vi "CSClassUtilities.InheritClass.vi"() -> ()   [LabVIEW 2014]
doc: "This tool allows one to inherit a class from a parent class.\n\nLicense Agreement for this software:\n\nCopyright (C) 2001 Dietrich Beck, Holger Brand, Mathias Richter\nGSI Helmholtzzentrum für Schwerionenforschung GmbH\nPlanckstraße 1\nD-64291 Darmstadt\nGermany\n\nContact: d.beck@gsi.de \n\nThis program is free software: you can redistribute it and/or modify it under the terms\nof the GNU General Public License as published by the Free Software Foundation, either\nversion 3 of the License, or (at your option) any later version.\n\nThis program is distributed in the hope that it will be useful, but WITHOUT ANY WARRANTY;\nwithout even the implied warranty of MERCHANTABILITY or FITNESS FOR A PARTICULAR PURPOSE. See the GNU General Public License for more details.\n\nYou should have received a copy of the GNU General Public License along with this program.\nIf not, see <http://www.gnu.org/licenses/>.\n\nFor all questions and ideas contact: d.beck@gsi.de\nLast update: 19-Nov-2010"
uses:
  CSClass/CSCore/CSSystem/CoreLib/CoreLib.lvlib
  CSClass/CSCore/CSSystem/CSSystemLib/CSSystemLib.lvlib
panel:
  in  "GUI":T1(tab)=enum."NewClass"
  in  "Continue1":bool
  in  "Continue2":bool
  in  "Select parent class":i32(listbox)
  in  "Continue3":bool
  in  "New class name":string
  in  "Select Class Group":i32(listbox)
  out "Done?":bool
  out "Parent Class":string
  out "New Class":string
  # "1) This tool  will open and rename a couple of VIs. It is strongly recommended to use this tool not from a project but directly after launching LabVIEW!\n\n2) This tool may overwrite existing VIs. It is recommended to back up the class directory structure.\n\n3) This tool will only work on classes that are below the \".../CSClass\" folder.\n\n4) Public and protected class methods of a class will not be re-created in the child class. If you would like to use such methods of a (grand-) parent class, use direct method calls. No copy and paste! As a consequence, this tool is not required for inheritance. The parent class of a child class is defined by calling the constructor of the parent class within the constructor of the child class (Of course, one should call the deconstructor of the parent class within the deconstructor of the child class).\n\n5) Only in exceptional cases, copies of methods must be created in a child class.  Examples are the constructor/destructor methods.. \n\nPLEASE CONTINUE ONLY, IF THIS VI HAS BEEN LOADED DIRECTLY AFTER LAUNCHING LabVIEW!"
  # "1) When done, it is recommended to exit and restart LabVIEW.\n\n2) It is good idea to refine the methods of the class created by \n     a) modifying the icons of the methods.\n     b) editing the attribute data (.../CLASSNAME/private/i attribute.ctl).\n     c) adding new functionality to the class."
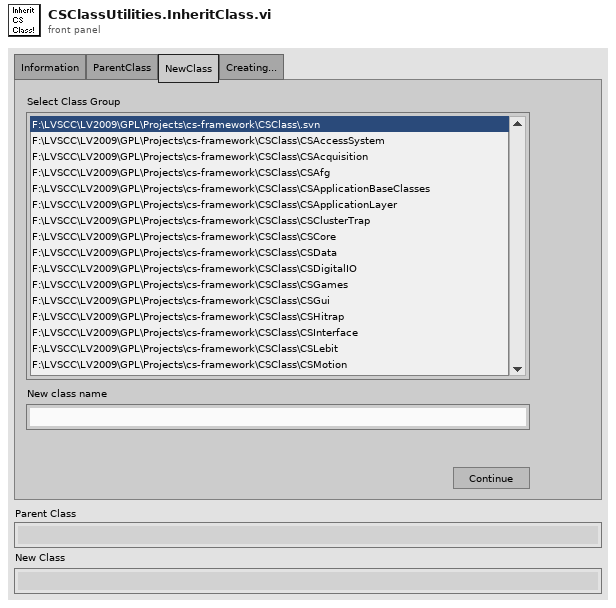
[diagram p1: front panel]
types:
  T1 = enum32{"Information", "ParentClass", "NewClass", "Creating..."}
  T2 = enum32{"invalid scope", "public", "private", "protected"}
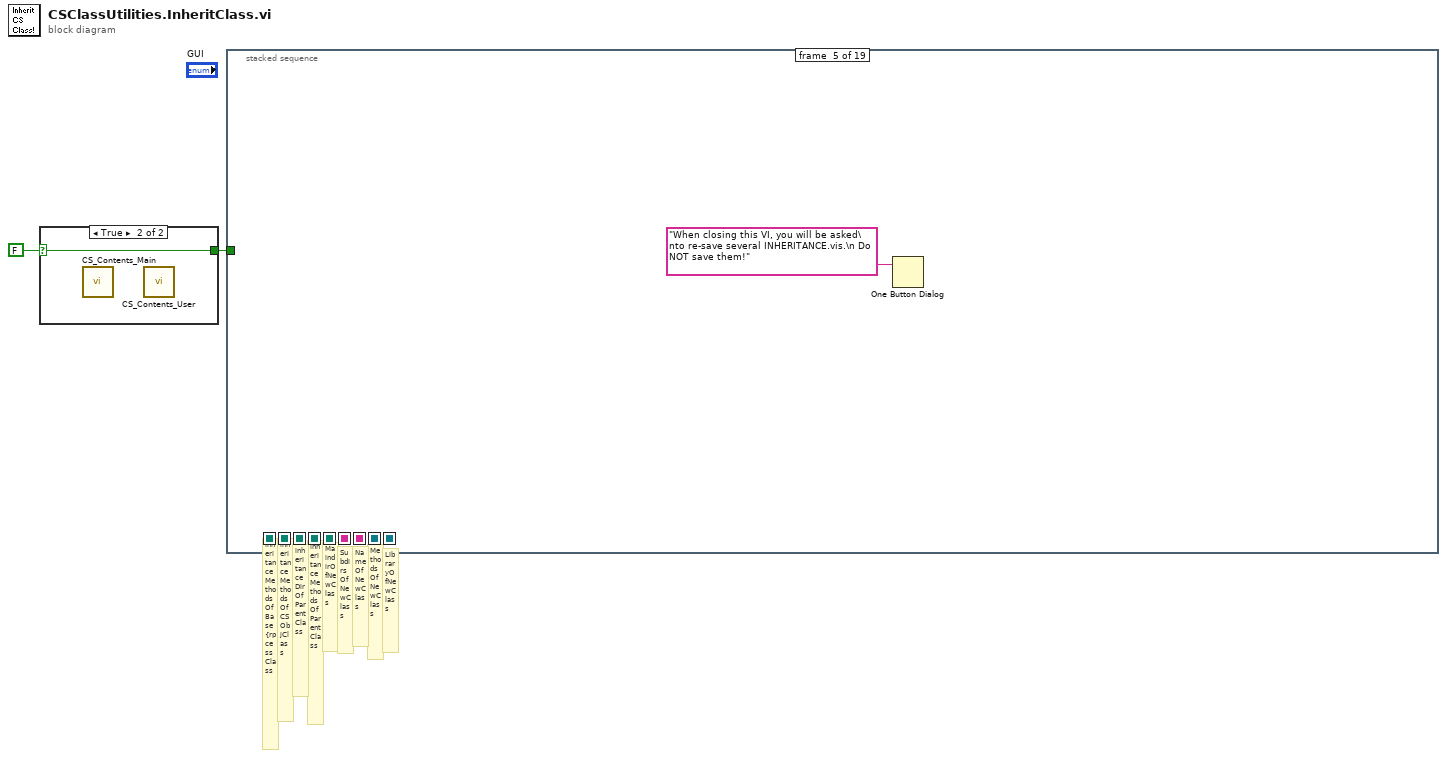
[diagram p0: block diagram]
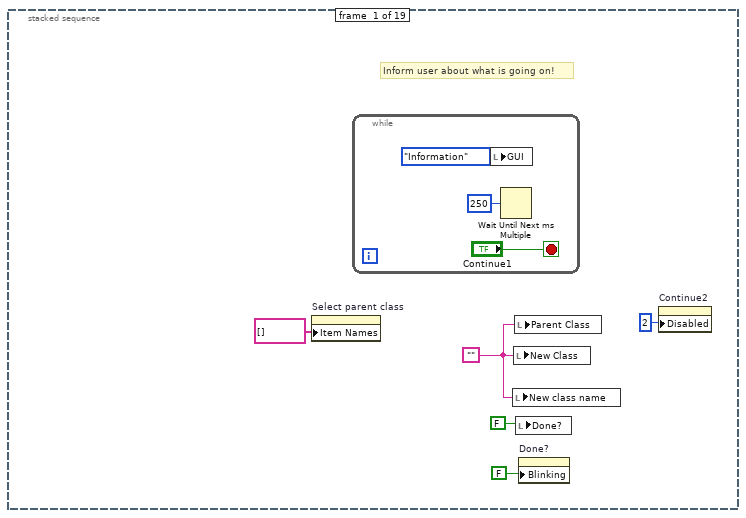
[diagram p3: hidden frame]
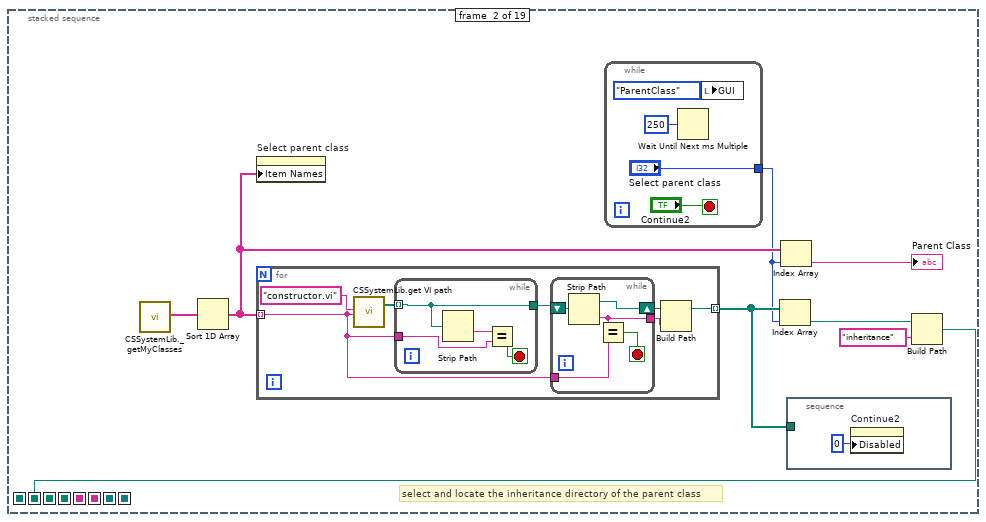
[diagram p4: hidden frame]
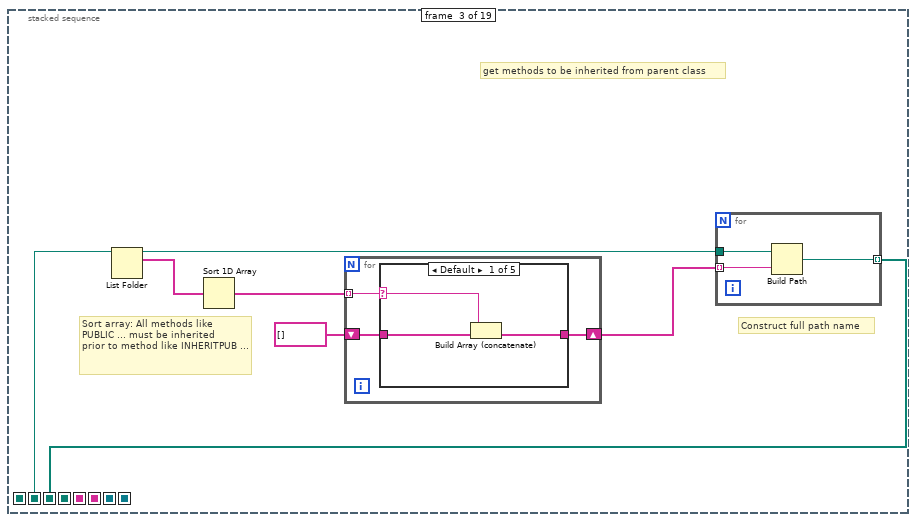
[diagram p5: hidden frame]
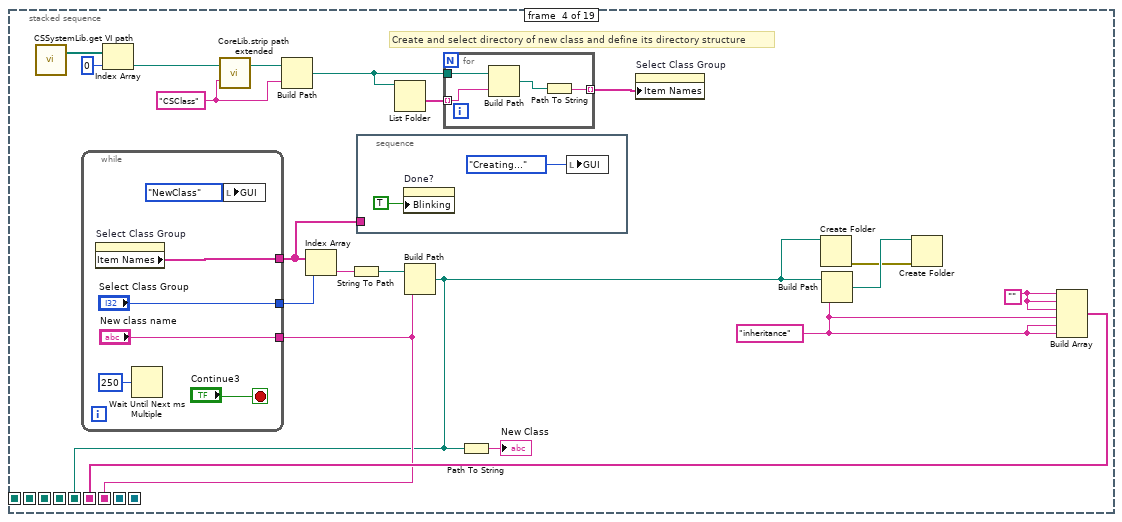
[diagram p10: hidden frame]
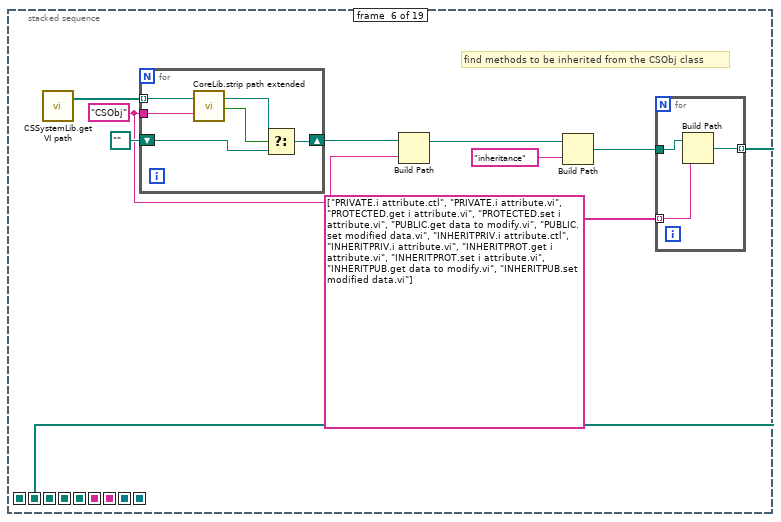
[diagram p11: hidden frame]
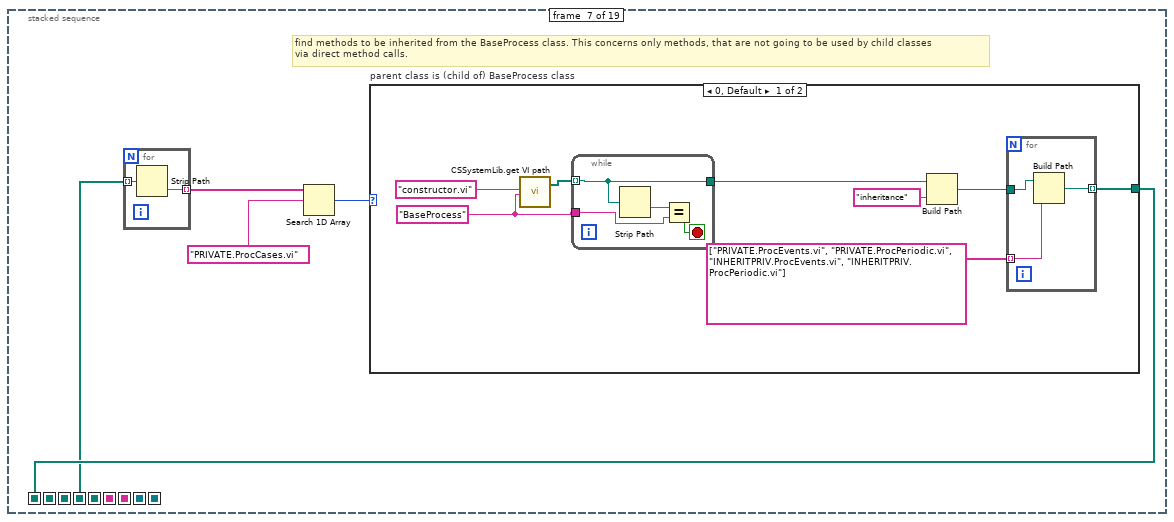
[diagram p12: hidden frame]
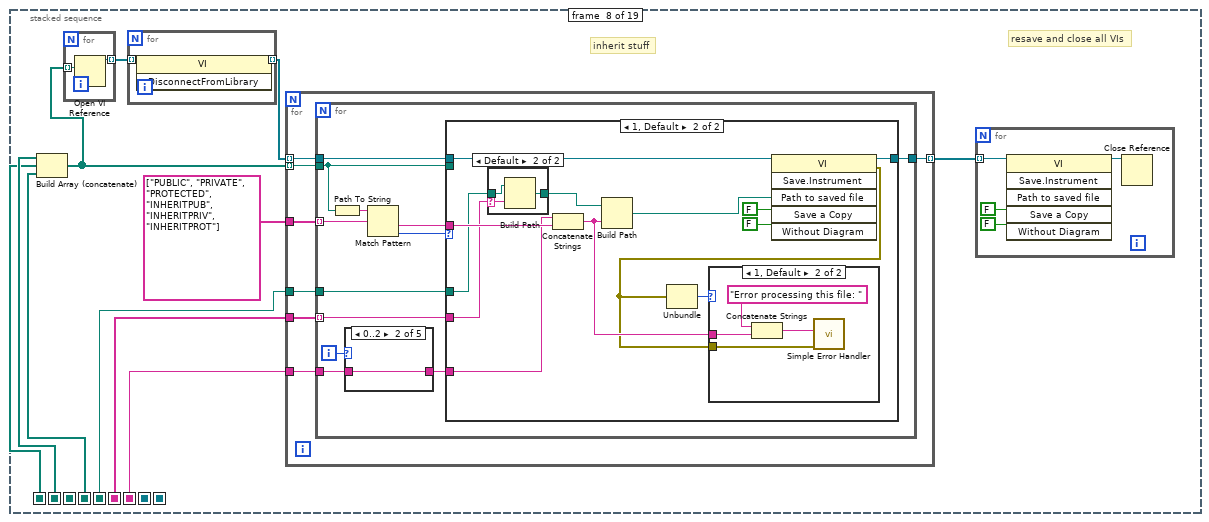
[diagram p14: hidden frame]
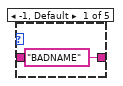
[diagram p15: hidden frame]
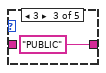
[diagram p16: hidden frame]
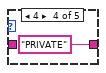
[diagram p17: hidden frame]
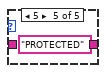
[diagram p18: hidden frame]
diagram:
  # "LibraryOfNewClass"
  # "MethodsOfNewClass"
  # "inheritanceMethodsOfBase{rpcessClass"
  # "inheritanceMethodsOfCSObjClass"
  # "NameOfNewClass"
  # "MaindirOfNewClass"
  # "SubdirsOfNewClass"
  # "inheritanceMethodsOfParentClass"
  # "inheritanceDirOfParentClass"
  n1 = case shown="True" FALSE {
    selector: FALSE -> [_ w3]
    tunnel: [_ w3] -> w1
    frame False {
    }
    frame True {
      n2 = call "CS_Contents_Main.vi"() -> ()  [unwired: 1 in]
      n3 = call "CS_Contents_User.vi"() -> ()  [unwired: 1 in]
    }
  }
  n4 = stacked-sequence {
    seq-local: [_ _ _ w67 _ _ _ _ _ _ _ _ _ _ _ _ _ _ _] -> [_ _ _ _ _ _ _ w144 _ _ _ _ w274 w305 w334 w362 w400 _ _]
    seq-local: [_ _ _ w77 _ _ _ _ _ _ _ _ _ _ _ _ _ _ _] -> [_ _ _ _ _ _ _ w143 _ _ _ _ _ _ _ _ _ _ _]
    seq-local: [_ w19 _ _ _ _ _ _ _ _ _ _ _ _ _ _ _ _ _] -> [_ _ w47 _ _ _ _ _ _ _ _ _ _ _ _ _ _ _ _]
    seq-local: [_ _ w44 _ _ _ _ _ _ _ _ _ _ _ _ _ _ _ _] -> [_ _ _ _ _ _ w114 w139 w200 w222 _ _ _ _ _ _ _ _ _]
    seq-local: [_ _ _ w66 _ _ _ _ _ _ _ _ _ _ _ _ _ _ _] -> [_ _ _ _ _ _ _ w134 w199 w221 w243 w260 w273 w304 w333 w361 w401 _ _]
    seq-local: [_ _ _ _ _ w97 _ _ _ _ _ _ _ _ _ _ _ _ _] -> [_ _ _ _ _ _ _ w140 _ _ _ _ _ _ _ _ _ _ _]
    seq-local: [_ _ _ _ _ _ w116 _ _ _ _ _ _ _ _ _ _ _ _] -> [_ _ _ _ _ _ _ w138 _ _ _ _ _ _ _ _ _ _ _]
    seq-local: [_ _ _ _ _ _ _ _ _ _ _ w250 _ _ _ _ _ _ _] -> [_ _ _ _ _ _ _ _ _ _ _ _ _ _ _ _ _ w403 _]
    seq-local: [_ _ _ _ _ _ _ _ _ _ _ _ w269 _ _ _ _ _ _] -> [_ _ _ _ _ _ _ _ _ _ _ _ _ w301 w330 w358 w394 _ _]
    tunnel: w1 -> [_ _ _ _ _ _ _ _ _ _ _ _ _ _ _ _ _ _ _]
    frame #0 {
      w6 = "" ("New class name")
      # "Inform user about what is going on!"
      n5 = property on="Select parent class" class="LstBox (strict)"("Item Names"=string[] []) -> ()  [unwired: 2 in, 2 out]
      n6 = while {
        stop <- "Continue1" stop-if-true
        n7 = local write "GUI"(T1."Information" ("GUI")) -> ()
        n8 = Wait Until Next ms Multiple(millisecond multiple=u32 250) -> ()  [unwired: 1 out]
      }
      n9 = local write "New class name"(w6) -> ()
      n10 = local write "New Class"(w6) -> ()
      n11 = local write "Parent Class"(w6) -> ()
      n12 = local write "Done?"(FALSE ("Done?")) -> ()
      n13 = property on="Done?" class="Bool (strict)"("Blinking"=FALSE) -> ()  [unwired: 2 in, 2 out]
      n14 = property on="Continue2" class="Bool"("Disabled"=u8 2) -> ()  [unwired: 2 in, 2 out]
    }
    frame #1 {
      # "select and locate the inheritance directory of the parent class"
      n15 = call "CSSystemLib._getMyClasses.vi"() -> ("myClasses"=w16:string[])  [unwired: 18 in, 1 out]
      n16 = Sort 1D Array(array=w16) -> (sorted array=w14:string[])
      n17 = property on="Select parent class" class="LstBox (strict)"("Item Names"=w14) -> ()  [unwired: 2 in, 2 out]
      n18 = for {
        tunnel: w14 -> [w20] mode=indexing
        tunnel: [w23] -> w15 mode=indexing
        n19 = call "CSSystemLib.get VI path.vi"("method"="constructor.vi" ("Method"), "class"=w20) -> ("Directories"=w22:path[])  [unwired: 15 in, 2 out]
        n20 = while {
          tunnel: w22 -> [w29] mode=indexing
          tunnel: [w29] -> w21
          tunnel: w20 -> [w28]
          stop <- w27 stop-if-true
          n21 = Strip Path(path=w29) -> (name=w30:string)  [unwired: 1 out]
          n22 = Equal?(x=w30, y=w28) -> (x = y?=w27:bool)
        }
        n23 = while {
          shift-right: [w34] -> w25
          shift-left: w21 -> [w35]
          tunnel: w20 -> [w33]
          tunnel: [w31] -> w24
          stop <- w32 stop-if-true
          n24 = Strip Path(path=w35) -> (stripped path=w34:path, name=w31:string)
          n25 = Equal?(x=w31, y=w33) -> (x = y?=w32:bool)
        }
        n26 = Build Path(base path=w25, name or relative path=w24) -> (appended path=w23:path)
      }
      n27 = while {
        tunnel: ["Select parent class"] -> w13
        stop <- "Continue2" stop-if-true
        n28 = Wait Until Next ms Multiple(millisecond multiple=u32 250) -> ()  [unwired: 1 out]
        n29 = local write "GUI"(T1."ParentClass" ("GUI")) -> ()
      }
      n30 = Index Array(array=w15, index=w13) -> (element=w17:path)
      n31 = Index Array(array=w14, index=w13) -> (element=→"Parent Class":string)
      n32 = stacked-sequence {
        tunnel: w15 -> [_]
        frame #0 {
          n33 = property on="Continue2" class="Bool"("Disabled"=u8 0) -> ()  [unwired: 2 in, 2 out]
        }
      }
      n34 = Build Path(base path=w17, name or relative path="inheritance") -> (appended path=w19:path)
    }
    frame #2 {
      # "get methods to be inherited from parent class"
      # "Construct full path name"
      # "Sort array: All methods like\nPUBLIC ... must be inherited\nprior to method like INHERITPUB ..."
      n35 = List Folder(path=w47) -> (path out=w45:path, filenames=w46:string[])  [unwired: 3 in, 2 out]
      n36 = Sort 1D Array(array=w46) -> (sorted array=w42:string[])
      n37 = for {
        tunnel: w42 -> [w50] mode=indexing
        shift-right: [w48] -> w41
        shift-left: string[] [] -> [w49]
        n38 = case shown="Default" w50 {
          selector: w50 -> [w51 _ _ _ _]
          tunnel: w49 -> [w53 w54 w55 w56 w57]
          tunnel: [w52 w54 w55 w56 w57] -> w48
          frame Default {
            n39 = Build Array (concatenate)(w51, w53) -> (w52:string[])
          }
          frame "PRIVATE.ProcEvents.vi" {
          }
          frame "PRIVATE.ProcPeriodic.vi" {
          }
          frame "INHERITPRIV.ProcEvents.vi" {
          }
          frame "INHERITPRIV.ProcPeriodic.vi" {
          }
        }
      }
      n40 = for {
        tunnel: w41 -> [w59] mode=indexing
        tunnel: w45 -> [w60]
        tunnel: [w58] -> w44 mode=indexing
        n41 = Build Path(base path=w60, name or relative path=w59) -> (appended path=w58:path)
      }
    }
    frame #3 {
      w62 = "" ("Empty String Constant")
      w63 = "inheritance"
      w71 = "CSClass" ("search string")
      # "Create and select directory of new class and define its directory structure"
      n42 = call "CSSystemLib.get VI path.vi"() -> ("Directories"=w79:path[])  [unwired: 17 in, 2 out]
      n43 = while {
        tunnel: [w90] -> w76
        tunnel: ["Select Class Group"] -> w78
        tunnel: ["New class name"] -> w67
        stop <- "Continue3" stop-if-true
        n44 = property on="Select Class Group" class="LstBox (strict)"() -> ("Item Names"=w90:string[])  [unwired: 2 in, 2 out]
        n45 = Wait Until Next ms Multiple(millisecond multiple=u32 250) -> ()  [unwired: 1 out]
        n46 = local write "GUI"(T1."NewClass" ("GUI")) -> ()
      }
      n47 = Index Array(array=w79, index=0) -> (element=w73:path)
      n48 = call "CoreLib.strip path extended.vi"("Path"=w73, "search string"=w71) -> ("stripped path"=w72:path)  [unwired: 15 in, 2 out]
      n49 = Build Path(base path=w72, name or relative path=w71) -> (appended path=w70:path)
      n50 = Index Array(array=w76, index=w78) -> (element=w69:string)
      n51 = String To Path(string=w69) -> (path=w68:path)
      n52 = stacked-sequence {
        tunnel: w76 -> [_]
        frame #0 {
          n53 = property on="Done?" class="Bool (strict)"("Blinking"=TRUE) -> ()  [unwired: 2 in, 2 out]
          n54 = local write "GUI"(T1."Creating..." ("GUI")) -> ()
        }
      }
      n55 = List Folder(path=w70) -> (folder names=w75:string[])  [unwired: 3 in, 3 out]
      n56 = Build Path(base path=w68, name or relative path=w67) -> (appended path=w66:path)
      n57 = for {
        tunnel: w75 -> [w83] mode=indexing
        tunnel: [w81] -> w74 mode=indexing
        tunnel: w70 -> [w84]
        n58 = Build Path(base path=w84, name or relative path=w83) -> (appended path=w82:path)
        n59 = Path To String(path=w82) -> (string=w81:string)
      }
      n60 = Path To String(path=w66) -> (string=→"New Class":string)
      n61 = property on="Select Class Group" class="LstBox (strict)"("Item Names"=w74) -> ()  [unwired: 2 in, 2 out]
      n62 = Create Folder(path (use dialog)=w66) -> (error out=w61:errorcluster)  [unwired: 2 in, 2 out]
      n63 = Build Path(base path=w66, name or relative path=w63) -> (appended path=w64:path)
      n64 = Create Folder(path (use dialog)=w64, error in=w61) -> ()  [unwired: 1 in, 3 out]
      n65 = Build Array(w62, w62, w62, w63, w63, w63) -> (w77:string[])
    }
    frame #4 {
      n66 = One Button Dialog(message="When closing this VI, you will be asked\nto re-save several INHERITANCE.vis.\n Do NOT save them!") -> ()  [unwired: 1 in, 1 out]
    }
    frame #5 {
      w95 = "CSObj" ("search string")
      # "find methods to be inherited from the CSObj class"
      n67 = call "CSSystemLib.get VI path.vi"() -> ("Directories"=w102:path[])  [unwired: 17 in, 2 out]
      n68 = for {
        tunnel: w102 -> [w111] mode=indexing
        shift-right: [w110] -> w96
        shift-left: path "" ("stripped path") -> [w107]
        tunnel: w95 -> [w106]
        n69 = call "CoreLib.strip path extended.vi"("Path"=w111, "search string"=w106) -> ("stripped path"=w108:path, "found?"=w109:bool)  [unwired: 15 in, 1 out]
        n70 = Select(t=w108, s=w109, f=w107) -> (s? t:f=w110:path)
      }
      n71 = Build Path(base path=w96, name or relative path=w95) -> (appended path=w94:path)
      n72 = Build Path(base path=w94, name or relative path="inheritance") -> (appended path=w98:path)
      n73 = for {
        tunnel: string[] ["PRIVATE.i attribute.ctl", "PRIVATE.i attribute.vi", "PROTECTED.get i attribute.vi", "PROTECTED.set i attribute.vi", "PUBLIC.get data to modify.vi", "PUBLIC.set modified data.vi", "INHERITPRIV.i attribute.ctl", "INHERITPRIV.i attribute.vi", "INHERITPROT.get i attribute.vi", "INHERITPROT.set i attribute.vi", "INHERITPUB.get data to modify.vi", "INHERITPUB.set modified data.vi"] -> [w104] mode=indexing
        tunnel: w98 -> [w105]
        tunnel: [w103] -> w97 mode=indexing
        n74 = Build Path(base path=w105, name or relative path=w104) -> (appended path=w103:path)
      }
    }
    frame #6 {
      # "find methods to be inherited from the BaseProcess class. This concerns only methods, that are not going to be used by child classes\nvia direct method calls."
      n75 = for {
        tunnel: w114 -> [w118] mode=indexing
        tunnel: [w117] -> w113 mode=indexing
        n76 = Strip Path(path=w118) -> (name=w117:string)  [unwired: 1 out]
      }
      n77 = Search 1D Array(1D array=w113, element="PRIVATE.ProcCases.vi" ("string")) -> (index of element=w115:i32)  [unwired: 1 in]
      n78 = case "parent class is (child of) BaseProcess class" shown="0, Default" w115 {
        tunnel: [w123 _] -> w116
        frame 0, Default {
          w119 = "BaseProcess" ("search string")
          n79 = call "CSSystemLib.get VI path.vi"("method"="constructor.vi" ("Method"), "class"=w119) -> ("Directories"=w120:path[])  [unwired: 15 in, 2 out]
          n80 = while {
            tunnel: w120 -> [w129] mode=indexing
            tunnel: [w129] -> w121
            tunnel: w119 -> [w128]
            stop <- w127 stop-if-true
            n81 = Strip Path(path=w129) -> (name=w130:string)  [unwired: 1 out]
            n82 = Equal?(x=w130, y=w128) -> (x = y?=w127:bool)
          }
          n83 = Build Path(base path=w121, name or relative path="inheritance") -> (appended path=w124:path)
          n84 = for {
            tunnel: string[] ["PRIVATE.ProcEvents.vi", "PRIVATE.ProcPeriodic.vi", "INHERITPRIV.ProcEvents.vi", "INHERITPRIV.ProcPeriodic.vi"] -> [w132] mode=indexing
            tunnel: w124 -> [w133]
            tunnel: [w131] -> w123 mode=indexing
            n85 = Build Path(base path=w133, name or relative path=w132) -> (appended path=w131:path)
          }
        }
        frame -1 {
        }
      }
    }
    frame #7 {
      # "inherit stuff"
      # "resave and close all VIs"
      n86 = Build Array (concatenate)(w140, w138, w139) -> (w136:path[])
      n87 = for {
        tunnel: w136 -> [w148] mode=indexing
        tunnel: [w147] -> w137 mode=indexing
        n88 = Open VI Reference(vi path=w148) -> (vi reference=w147:refnum<vi>)  [unwired: 5 in, 1 out]
      }
      n89 = for {
        tunnel: w137 -> [w146] mode=indexing
        tunnel: [w145] -> w135 mode=indexing
        n90 = invoke on="Invoke Node" class="VI" method="DisconnectFromLibrary"(reference=w146) -> (reference out=w145:refnum<vi>)  [unwired: 2 in, 2 out]
      }
      n91 = for {
        tunnel: string[] ["PUBLIC", "PRIVATE", "PROTECTED", "INHERITPUB", "INHERITPRIV", "INHERITPROT"] -> [w159]
        tunnel: w144 -> [w158]
        tunnel: w134 -> [w157]
        tunnel: w143 -> [w156]
        tunnel: w136 -> [w155] mode=indexing
        tunnel: [w154] -> w141 mode=indexing
        tunnel: w135 -> [w153] mode=indexing
        n92 = for {
          tunnel: w159 -> [w171] mode=indexing
          tunnel: w158 -> [w166]
          tunnel: w157 -> [w170]
          tunnel: w156 -> [w168] mode=indexing
          tunnel: w155 -> [w162]
          tunnel: w153 -> [w160]
          tunnel: [w161] -> w154
          i -> [w164]
          n93 = Path To String(path=w162) -> (string=w163:string)
          n94 = case shown="0..2" w164 {
            tunnel: ["BADNAME" w173 "PUBLIC" "PRIVATE" "PROTECTED"] -> w165
            tunnel: w166 -> [_ w173 _ _ _]
            frame -1, Default {
            }
            frame 0..2 {
            }
            frame 3 {
            }
            frame 4 {
            }
            frame 5 {
            }
          }
          n95 = Match Pattern(string=w163, regular expression=w171) -> (after substring=w169:string, offset past match=w167:i32)  [unwired: 1 in, 2 out]
          n96 = case shown="1, Default" w167 {
            tunnel: w169 -> [_ w190]
            tunnel: w165 -> [_ w189]
            tunnel: w170 -> [_ w186]
            tunnel: w168 -> [_ w179]
            tunnel: w162 -> [_ _]
            tunnel: [w177 w182] -> w161
            tunnel: w160 -> [w177 w178]
            frame -1 {
            }
            frame 1, Default {
              n97 = case shown="Default" w179 {
                selector: w179 -> [_ w192]
                tunnel: w186 -> [w191 w194]
                tunnel: [w191 w193] -> w185
                frame "" {
                }
                frame Default {
                  n98 = Build Path(base path=w194, name or relative path=w192) -> (appended path=w193:path)
                }
              }
              n99 = Concatenate Strings(w189, w190) -> (w184:string)
              n100 = Build Path(base path=w185, name or relative path=w184) -> (appended path=w183:path)
              n101 = invoke on="Invoke Node" class="VI" method="Save.Instrument"(reference=w178, "Path to saved file"=w183, "Save a Copy"=FALSE, "Without Diagram"=FALSE) -> (reference out=w182:refnum<vi>, error out=w180:errorcluster)  [unwired: 2 in, 4 out]
              n102 = Unbundle(w180) -> ("code"=w181:i32)  [unwired: 2 out]
              n103 = case shown="1, Default" w181 {
                tunnel: w184 -> [_ w198]
                tunnel: w180 -> [_ w195]
                frame 0, 1051 {
                }
                frame 1, Default {
                  n104 = Concatenate Strings("Error processing this file: ", w198) -> (w196:string)
                  n105 = call <vilib>:"Simple Error Handler.vi"("error source (\" \")"=w196, "error in (no error)"=w195) -> ()  [unwired: 3 in, 5 out]
                }
              }
            }
          }
        }
      }
      n106 = for {
        tunnel: w141 -> [w151] mode=indexing
        n107 = invoke on="Invoke Node" class="VI" method="Save.Instrument"(reference=w151, "Save a Copy"=FALSE, "Without Diagram"=FALSE) -> (reference out=w152:refnum<vi>)  [unwired: 3 in, 5 out]
        n108 = Close Reference(reference=w152) -> ()  [unwired: 1 in, 1 out]
      }
    }
    frame #8 {
      # "prepare inheritance for the next generation"
      n109 = disable-structure "Diagram Disable Structure" shown="Disabled" {
        disable-tunnel: w200 -> [w202 _]
        disable-tunnel: w199 -> [w201 _]
        frame Disabled {
          # "I think this does not work anymore, since the inheritance VIs know from which library they are"
          n110 = for {
            tunnel: string[] ["INHERITPUB", "INHERITPRIV", "INHERITPROT"] -> [w206]
            tunnel: w201 -> [w205]
            tunnel: w202 -> [w204] mode=indexing
            n111 = for {
              tunnel: w206 -> [w207] mode=indexing
              tunnel: w205 -> [w212]
              tunnel: w204 -> [w208]
              n112 = Path To String(path=w208) -> (string=w209:string)
              n113 = Match Pattern(string=w209, regular expression=w207) -> (after substring=w211:string, offset past match=w210:i32)  [unwired: 1 in, 2 out]
              n114 = case shown="1, Default" w210 {
                tunnel: w211 -> [_ w220]
                tunnel: w207 -> [_ w219]
                tunnel: w212 -> [_ w217]
                tunnel: w208 -> [_ w218]
                frame -1 {
                }
                frame 1, Default {
                  n115 = Build Path(base path=w217, name or relative path="inheritance") -> (appended path=w216:path)
                  n116 = Concatenate Strings(w219, w220) -> (w215:string)
                  n117 = Build Path(base path=w216, name or relative path=w215) -> (appended path=w214:path)
                  n118 = Copy(10:w214, 11:w218) -> ()  [unwired: 3 in, 3 out]
                }
              }
            }
          }
        }
        frame Enabled {
        }
      }
    }
    frame #9 {
      n119 = disable-structure "Diagram Disable Structure" shown="Disabled" {
        disable-tunnel: w222 -> [w225 _]
        disable-tunnel: w221 -> [w223 _]
        frame Disabled {
          w224 = string[] ["INHERITPRIV.ProcCases.vi", "INHERITPRIV.ProcState.vi"]  # exception list
          # "I think this does not work anymore, since the inheritance VIs know from which library they are"
          # "prepare inheritance for the next generation: We must overwrite VIs of the exception list.\nAll methods that have no link to a method of the direct parent class must be included here."
          n120 = for {
            tunnel: w224 -> [w228]
            tunnel: w223 -> [w227]
            tunnel: w225 -> [w226] mode=indexing
            n121 = for {
              tunnel: w228 -> [w229] mode=indexing
              tunnel: w227 -> [w234]
              tunnel: w226 -> [w230]
              n122 = Path To String(path=w230) -> (string=w231:string)
              n123 = Match Pattern(string=w231, regular expression=w229) -> (after substring=w233:string, offset past match=w232:i32)  [unwired: 1 in, 2 out]
              n124 = case shown="1, Default" w232 {
                tunnel: w233 -> [_ w242]
                tunnel: w229 -> [_ w241]
                tunnel: w234 -> [_ w239]
                tunnel: w230 -> [_ w240]
                frame -1 {
                }
                frame 1, Default {
                  n125 = Build Path(base path=w239, name or relative path="inheritance") -> (appended path=w236:path)
                  n126 = Concatenate Strings(w241, w242) -> (w237:string)
                  n127 = Build Path(base path=w236, name or relative path=w237) -> (appended path=w235:path)
                  n128 = Copy(10:w235, 11:w240) -> ()  [unwired: 3 in, 3 out]
                }
              }
            }
          }
        }
        frame Enabled {
        }
      }
    }
    frame #10 {
      # "delete some methods inherited from the (grand) parent classes, that next generation classes will get directly from (grand) parents."
      n129 = Build Path(base path=w243, name or relative path="inheritance") -> (appended path=w244:path)
      n130 = for {
        tunnel: string[] ["PRIVATE.i attribute.ctl", "PRIVATE.i attribute.vi", "PROTECTED.get i attribute.vi", "PROTECTED.set i attribute.vi", "PUBLIC.get data to modify.vi", "PUBLIC.set modified data.vi", "INHERITPRIV.i attribute.ctl", "INHERITPRIV.i attribute.vi", "INHERITPROT.get i attribute.vi", "INHERITPROT.set i attribute.vi", "INHERITPUB.get data to modify.vi", "INHERITPUB.set modified data.vi", "PRIVATE.ProcEvents.vi", "PRIVATE.ProcPeriodic.vi", "INHERITPRIV.ProcEvents.vi", "INHERITPRIV.ProcPeriodic.vi"] -> [w248] mode=indexing
        tunnel: w244 -> [w249]
        n131 = Build Path(base path=w249, name or relative path=w248) -> (appended path=w247:path)
        n132 = Delete(path (use dialog)=w247) -> ()  [unwired: 4 in, 3 out]
      }
    }
    frame #11 {
      # "get names of all VIs"
      n133 = Build Path(base path=w260, name or relative path="inheritance") -> (appended path=w258:path)
      n134 = List Folder(path=w258) -> (path out=w257:path, filenames=w256:string[])  [unwired: 3 in, 2 out]
      n135 = List Folder(path=w260) -> (path out=w255:path, filenames=w254:string[])  [unwired: 3 in, 2 out]
      n136 = for {
        tunnel: w257 -> [w268]
        tunnel: w256 -> [w267] mode=indexing
        tunnel: [w266] -> w252 mode=indexing
        n137 = Build Path(base path=w268, name or relative path=w267) -> (appended path=w266:path)
      }
      n138 = for {
        tunnel: w255 -> [w265]
        tunnel: w254 -> [w264] mode=indexing
        tunnel: [w263] -> w253 mode=indexing
        n139 = Build Path(base path=w265, name or relative path=w264) -> (appended path=w263:path)
      }
      n140 = Build Array (concatenate)(w252, w253) -> (w251:path[])
      n141 = for {
        tunnel: w251 -> [w262] mode=indexing
        tunnel: [w261] -> w250 mode=indexing
        n142 = Open VI Reference(vi path=w262) -> (vi reference=w261:refnum<vi>)  [unwired: 5 in, 1 out]
      }
    }
    frame #12 {
      # "put public methods to library folder"
      n143 = invoke on="Invoke Node" class="App" method="Library.Create"() -> (error out=w277:errorcluster, "Create Library"=w279:refnum<vi>)  [unwired: 4 in, 2 out]
      n144 = invoke on="Invoke Node" class="Library" method="AddItem"(reference=w279, error in=w277, "Name"="public", "Path"=path "" ("Not A Path Constant"), "Type"="Folder") -> (reference out=w270:refnum<vi>, "AddItem"=w275:refnum<vi>)  [unwired: 1 in, 4 out]
      n145 = for {
        N: 4 -> [_]
        tunnel: w275 -> [w290]
        tunnel: w274 -> [w287]
        tunnel: w273 -> [w286]
        tunnel: [w282] -> w272
        i -> [w289]
        n146 = case shown="0, Default" w289 {
          tunnel: [".constructor.vi" ".destructor.vi" ".get data to modify.vi" ".set modified data.vi"] -> w288
          frame 0, Default {
          }
          frame 1 {
          }
          frame 2 {
          }
          frame 3 {
          }
        }
        n147 = Concatenate Strings(w287, w288) -> (w285:string)
        n148 = Build Path(base path=w286, name or relative path=w285) -> (appended path=w284:path)
        n149 = Not A Number/Path/Refnum?(number/path/refnum=w284) -> (NaN/Path/Refnum?=w283:bool)
        n150 = case "path does not exist?" shown="False" w283 {
          tunnel: w290 -> [w295 w296]
          tunnel: w285 -> [w294 _]
          tunnel: w284 -> [w292 _]
          tunnel: [w291 w296] -> w282
          frame False {
            n151 = invoke on="Invoke Node" class="ProjectItem" method="AddItem"(reference=w295, "Name"=w294, "Path"=w292, "Type"="VI") -> (reference out=w291:refnum<vi>)  [unwired: 2 in, 5 out]
          }
          frame True {
          }
        }
      }
      n152 = invoke on="Invoke Node" class="Library" method="Set Source Scope"(reference=w270, "SourceRef"=w272, "Scope"=T2."public" ("scope")) -> (reference out=w269:refnum<vi>)  [unwired: 2 in, 4 out]
    }
    frame #13 {
      # "put protected methods to library folder"
      n153 = invoke on="Invoke Node" class="Library" method="AddItem"(reference=w301, "Name"="protected", "Path"=path "" ("Not A Path Constant"), "Type"="Folder") -> ("AddItem"=w306:refnum<vi>)  [unwired: 2 in, 5 out]
      n154 = for {
        N: 4 -> [_]
        tunnel: w306 -> [w319]
        tunnel: w305 -> [w318]
        tunnel: w304 -> [w317]
        tunnel: [w311] -> w302
        i -> [w312]
        n155 = case shown="3" w312 {
          tunnel: [".get i attribute.vi" ".set i attribute.vi" ".ProcCases.vi" ".ProcPeriodic.vi"] -> w313
          frame 0, Default {
          }
          frame 1 {
          }
          frame 2 {
          }
          frame 3 {
          }
        }
        n156 = Concatenate Strings(w318, w313) -> (w316:string)
        n157 = Build Path(base path=w317, name or relative path=w316) -> (appended path=w315:path)
        n158 = Not A Number/Path/Refnum?(number/path/refnum=w315) -> (NaN/Path/Refnum?=w314:bool)
        n159 = case "path does not exist?" shown="False" w314 {
          tunnel: w319 -> [w328 w329]
          tunnel: w316 -> [w327 _]
          tunnel: w315 -> [w325 _]
          tunnel: [w324 w329] -> w311
          frame False {
            n160 = invoke on="Invoke Node" class="ProjectItem" method="AddItem"(reference=w328, "Name"=w327, "Path"=w325, "Type"="VI") -> (reference out=w324:refnum<vi>)  [unwired: 2 in, 5 out]
          }
          frame True {
          }
        }
      }
      n161 = invoke on="Invoke Node" class="Library" method="Set Source Scope"(reference=w301, "SourceRef"=w302, "Scope"=T2."public" ("scope")) -> ()  [unwired: 2 in, 5 out]
    }
    frame #14 {
      # "put private methods to library folder"
      n162 = invoke on="Invoke Node" class="Library" method="AddItem"(reference=w330, "Name"="private", "Path"=path "" ("Not A Path Constant"), "Type"="Folder") -> ("AddItem"=w335:refnum<vi>)  [unwired: 2 in, 5 out]
      n163 = for {
        N: 3 -> [_]
        tunnel: w335 -> [w348]
        tunnel: w334 -> [w347]
        tunnel: w333 -> [w346]
        tunnel: [w340] -> w331
        i -> [w341]
        n164 = case shown="2" w341 {
          tunnel: [".i attribute.ctl" ".i attribute.vi" ".ProcEvents.vi"] -> w342
          frame 0, Default {
          }
          frame 1 {
          }
          frame 2 {
          }
        }
        n165 = Concatenate Strings(w347, w342) -> (w345:string)
        n166 = Build Path(base path=w346, name or relative path=w345) -> (appended path=w344:path)
        n167 = Not A Number/Path/Refnum?(number/path/refnum=w344) -> (NaN/Path/Refnum?=w343:bool)
        n168 = case "path does not exist?" shown="True" w343 {
          tunnel: w348 -> [w356 w357]
          tunnel: w345 -> [w355 _]
          tunnel: w344 -> [w353 _]
          tunnel: [w352 w357] -> w340
          frame False {
            n169 = invoke on="Invoke Node" class="ProjectItem" method="AddItem"(reference=w356, "Name"=w355, "Path"=w353, "Type"="VI") -> (reference out=w352:refnum<vi>)  [unwired: 2 in, 5 out]
          }
          frame True {
          }
        }
      }
      n170 = invoke on="Invoke Node" class="Library" method="Set Source Scope"(reference=w330, "SourceRef"=w331, "Scope"=T2."private" ("scope")) -> ()  [unwired: 2 in, 5 out]
    }
    frame #15 {
      # "put stuff dedicated for inheritance to library folder"
      n171 = invoke on="Invoke Node" class="Library" method="AddItem"(reference=w358, "Name"="inheritance", "Path"=path "" ("Not A Path Constant"), "Type"="Folder") -> ("AddItem"=w363:refnum<vi>)  [unwired: 2 in, 5 out]
      n172 = for {
        N: 11 -> [_]
        tunnel: w363 -> [w376]
        tunnel: w362 -> [_]
        tunnel: w361 -> [w371]
        tunnel: [w368] -> w359
        i -> [w373]
        n173 = case shown="3" w373 {
          tunnel: ["INHERITPRIV.ProcCases.vi" "INHERITPRIV.ProcEvents.vi" "INHERITPRIV.ProcPeriodic.vi" "INHERITPUB.constructor.vi" "INHERITPUB.destructor.vi" "PRIVATE.ProcCases.vi" "PRIVATE.ProcEvents.vi" "PRIVATE.ProcPeriodic.vi" "PUBLIC.constructor.vi" "PUBLIC.destructor.vi" "PRIVATE.ProcState.vi"] -> w372
          frame 0, Default {
          }
          frame 1 {
          }
          frame 2 {
          }
          frame 3 {
          }
          frame 4 {
          }
          frame 5 {
          }
          frame 6 {
          }
          frame 7 {
          }
          frame 8 {
          }
          frame 9 {
          }
          frame 10 {
          }
        }
        n174 = Build Path(base path=w371, name or relative path="inheritance") -> (appended path=w370:path)
        n175 = Build Path(base path=w370, name or relative path=w372) -> (appended path=w375:path)
        n176 = Not A Number/Path/Refnum?(number/path/refnum=w375) -> (NaN/Path/Refnum?=w374:bool)
        n177 = case "path does not exist?" shown="False" w374 {
          tunnel: w376 -> [w392 w393]
          tunnel: w372 -> [w391 _]
          tunnel: w375 -> [w389 _]
          tunnel: [w388 w393] -> w368
          frame False {
            n178 = invoke on="Invoke Node" class="ProjectItem" method="AddItem"(reference=w392, "Name"=w391, "Path"=w389, "Type"="VI") -> (reference out=w388:refnum<vi>)  [unwired: 2 in, 5 out]
          }
          frame True {
          }
        }
      }
      n179 = invoke on="Invoke Node" class="Library" method="Set Source Scope"(reference=w358, "SourceRef"=w359, "Scope"=T2."public" ("scope")) -> ()  [unwired: 2 in, 5 out]
    }
    frame #16 {
      n180 = Concatenate Strings(w400, ".lvlib" ("string")) -> (w396:string)
      n181 = Build Path(base path=w401, name or relative path=w396) -> (appended path=w399:path)
      n182 = invoke on="Invoke Node" class="Library" method="Save"(reference=w394, "Path"=w399) -> (reference out=w398:refnum<vi>, error out=w397:errorcluster)  [unwired: 2 in, 2 out]
      n183 = Close Reference(reference=w398, error in (no error)=w397) -> ()  [unwired: 1 out]
    }
    frame #17 {
      # "save VIs of library"
      n184 = for {
        tunnel: w403 -> [w407] mode=indexing
        tunnel: [w405] -> w402 mode=indexing
        n185 = invoke on="Invoke Node" class="VI" method="Save.Instrument"(reference=w407, "Save a Copy"=FALSE) -> (reference out=w405:refnum<vi>)  [unwired: 4 in, 5 out]
      }
      n186 = for {
        tunnel: w402 -> [w404] mode=indexing
        n187 = Close Reference(reference=w404) -> ()  [unwired: 1 in, 1 out]
      }
    }
    frame #18 {
      n188 = One Button Dialog(message="Please do the following steps.\n1. Close and restart LabVIEW\n2. Add the lvlib-file of the new class to your project\n3. Open the VIs in the inheritance folders.\n4. Fix broken VIs\n5. You may have to replace a few inheritance VIs ") -> ()  [unwired: 1 in, 1 out]
      n189 = property on="Done?" class="Bool (strict)"("Blinking"=FALSE) -> ()  [unwired: 2 in, 2 out]
      "Done?" <- TRUE ("Done?")
    }
  }
